vi "I2C Write.vi"() -> ()   [LabVIEW 2020, in "CTI-Scratchpad.lvlib"]
uses:
  CTI-Scratchpad.lvlib
  CTI/I2C Number.ctl
  CTI/GPIO Number.ctl
  CTI/I2C Address.ctl
  CTI/Session/Session.lvclass
  CTI/VisaComms/VisaComms.lvclass
  CTI/CTI.lvlib
panel:
  in  "Data":string
  in  "Address":T1 format="%02x"
  in  "SDA GPIO":T2
  in  "SCL GPIO":T2
  in  "Baud":u32
  in  "I2C #":T3
  out "error out":errorcluster
  in  "Port":refnum<visa-resource-name>="COM7"
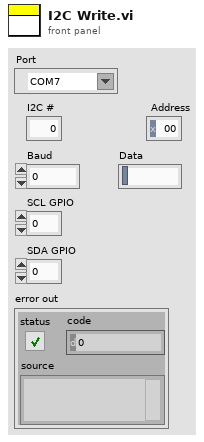
[diagram p1: front panel]
types:
  T1 = typedef "CTI.lvlib/I2C Address.ctl" = u8
  T2 = typedef "CTI.lvlib/GPIO Number.ctl" = i8
  T3 = typedef "CTI.lvlib/I2C Number.ctl" = i8
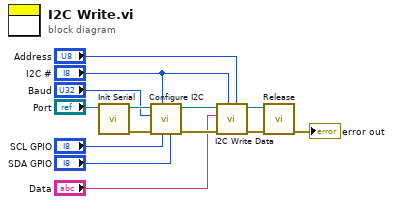
[diagram p0: block diagram]
diagram:
  n1 = call "Init Serial.vi"("VISA resource name in"="Port") -> ("error out"=w13:errorcluster, "Session"=w12:refnum<class "Session.lvclass">)  [unwired: 8 in, 1 out]
  n2 = call "Configure I2C.vi"("SDA GPIO"="SDA GPIO", "SCL GPIO"="SCL GPIO", "I2C #"="I2C #", "error in (no error)"=w13, "Baud"="Baud", "Session in"=w12) -> ("error out"=w11:errorcluster, "Session out"=w2:refnum<class "Session.lvclass">)  [unwired: 4 in]
  n3 = call "I2C Write Data.vi"("Address"="Address", "I2C #"="I2C #", "error in (no error)"=w11, "Data"="Data", "Session in"=w2) -> ("error out"=w10:errorcluster, "Session out"=w9:refnum<class "Session.lvclass">)  [unwired: 5 in]
  n4 = call-dynamic "Release.vi"("error in (no error)"=w10, "Session in"=w9) -> ("error out"=→"error out":errorcluster)  [unwired: 9 in]
